vi "Hatch Control.vi"(10 "Driver Right Bumper":bool, 11 "Driver Left Bumper":bool) -> (3 "Hatch Intake Floor":dbl)   [LabVIEW 2018]
uses:
  Infrastructure/Constants.vi
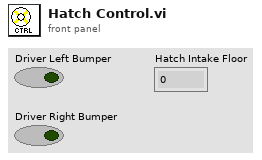
[diagram p1: front panel]
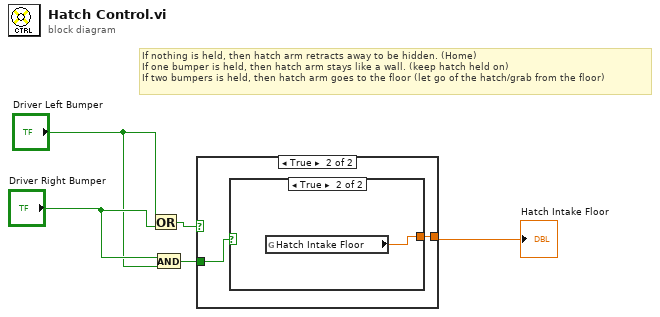
[diagram p0: block diagram]
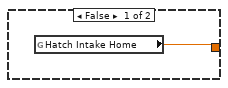
[diagram p2: hidden frame]
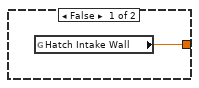
[diagram p3: hidden frame]
diagram:
  # "If nothing is held, then hatch arm retracts away to be hidden. (Home)\nIf one bumper is held, then hatch arm stays like a wall. (keep hatch held on)\nIf two bumpers is held, then hatch arm goes to the floor (let go of the hatch/grab from the floor)"
  n1 = Or(x="Driver Left Bumper", y="Driver Right Bumper") -> (x .or. y?=w1:bool)
  n2 = And(x="Driver Right Bumper", y="Driver Left Bumper") -> (x .and. y?=w2:bool)
  n3 = case shown="True" w1 {
    tunnel: w2 -> [_ w8]
    tunnel: [w6 w7] -> w3
    frame False {
      n4 = global read "Constants.vi" "Hatch Intake Home"() -> (w6:dbl)
    }
    frame True {
      n5 = case shown="True" w8 {
        tunnel: [w9 w10] -> w7
        frame False {
          n6 = global read "Constants.vi" "Hatch Intake Wall"() -> (w9:dbl)
        }
        frame True {
          n7 = global read "Constants.vi" "Hatch Intake Floor"() -> (w10:dbl)
        }
      }
    }
  }
  "Hatch Intake Floor" <- w3
